vi "Fluke7320.vi"() -> ()   [LabVIEW 2017]
uses:
  <vilib>/Instr/_visa.llb/VISA Configure Serial Port (Instr).vi
panel:
  out "output cluster":cluster{dbl}={9.99}
  in  "Tab Control":enum32{"Com Settings", "File"}(tab)
  in  "VISA resource name":refnum<visa-resource-name>="COM28"
  in  "baud rate 2":u32=2400
  in  "base path":path=path "E:/Materials Testing"
  in  "Filename":string="Run1_Fluke"
  out "file path":path=path "E:/Materials Testing/2018-04-16/Run4_Fluke.tdms"
  out "XY Graph":cluster{timestamp[], dbl[]}(graph)={[timestamp(3606762406.9225206 s since 1904-01-01)], [9.99]}
  out "Current Set":string="set:   10.00 C\r"
  in  "Update set?":bool
  in  "Set to":dbl=20.0 format="%#_13g"
  out "Heater Power":string="po:   20\r"
  out "Temperature":string="t:    9.99 C\r"
  out "error out":errorcluster
  in  "error in (no error)":errorcluster
  in  "Stop":bool
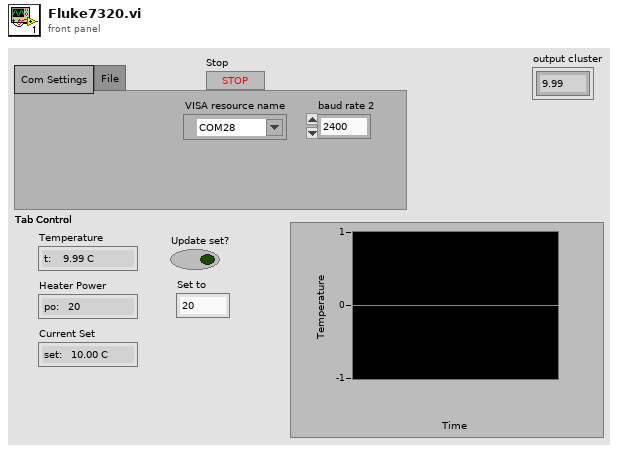
[diagram p1: front panel]
types:
  T1 = enum16{"open", "open or create", "create or replace", "create", "open (read-only)"}
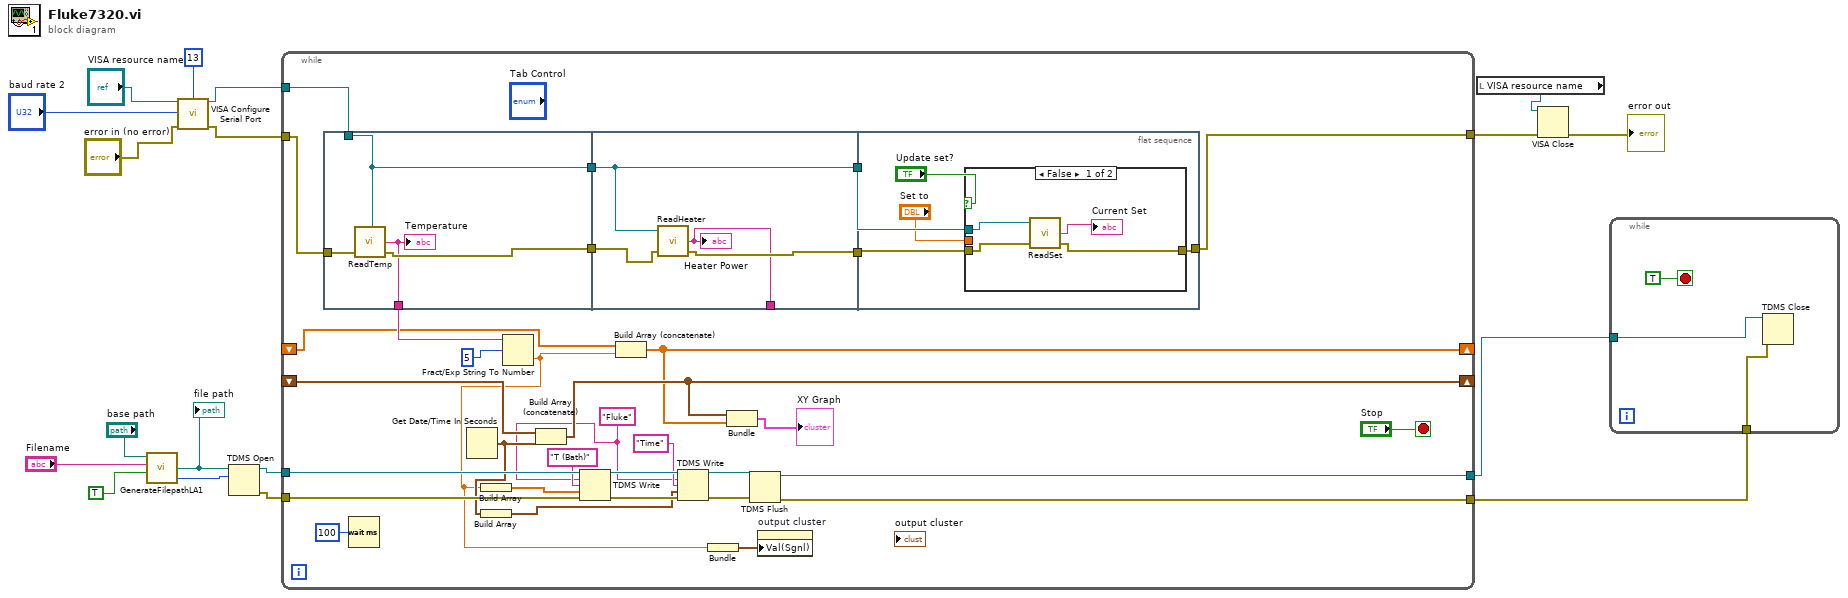
[diagram p0: block diagram]
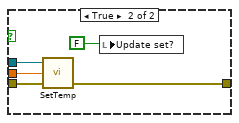
[diagram p2: hidden frame]
diagram:
  n1 = call "GenerateFilepathLA1.vi"("Auto Date folder"=TRUE, "Filename"="Filename", "base path"="base path") -> ("operation (0:open)"=w6:T1, "file path"=w5:path)  [unwired: 1 in, 1 out]
  "file path" <- w5
  n2 = call-poly "VISA Configure Serial Port"("VISA resource name"="VISA resource name", "termination char\n(0xA = '\\n' = LF)"=u8 13 ("termination char\n(0xA = '\\n' = LF)"), "baud rate (9600)"="baud rate 2", "error in (no error)"="error in (no error)") -> ("VISA resource name out"=w15:refnum<visa-resource-name>, "error out"=w14:errorcluster)  [unwired: 10 in]
  n3 = TDMS Open(10:w6, 11:w5) -> (0:w3:errorcluster, 3:w4:refnum<k34>)  [unwired: 5 in]
  n4 = while {
    tunnel: w14 -> [w48]
    tunnel: w15 -> [w47]
    tunnel: [w42] -> w10
    shift-right: [w36] -> _
    shift-left: _ -> [w39]
    shift-right: [w37] -> _
    shift-left: _ -> [w38]
    tunnel: w4 -> [w33]
    tunnel: w3 -> [w32]
    tunnel: [w25] -> w2
    tunnel: [w24] -> w1
    stop <- "Stop" stop-if-true
    w21 = "Fluke"
    n5 = flat-sequence {
      tunnel: w48 -> [w54]
      tunnel: w47 -> [w53]
      tunnel: [w53] -> w46
      tunnel: [w52] -> w45
      tunnel: [w51] -> w40
      tunnel: [w56] -> w44
      tunnel: w46 -> [w58]
      tunnel: [w58] -> w43
      tunnel: w45 -> [w57]
      tunnel: [w55] -> _
      tunnel: w44 -> [w63]
      tunnel: w43 -> [w62]
      tunnel: [w60] -> w42
      frame #0 {
        n6 = call "ReadTemp.vi"("error in (no error)"=w54, "VISA resource name"=w53) -> ("error out"=w52:errorcluster, "Temperature"=w51:string)  [unwired: 2 in]
        "Temperature" <- w51
      }
      frame #1 {
        n7 = call "ReadHeater.vi"("error in (no error)"=w57, "VISA resource name"=w58) -> ("error out"=w56:errorcluster, "Power"=w55:string)  [unwired: 1 in, 1 out]
        "Heater Power" <- w55
      }
      frame #2 {
        n8 = case shown="False" "Update set?" {
          tunnel: w63 -> [w66 w72]
          tunnel: [w65 w71] -> w60
          tunnel: w62 -> [w67 w70]
          tunnel: "Set to" -> [_ w69]
          frame False {
            n9 = call "ReadSet.vi"("error in (no error)"=w66, "VISA resource name"=w67) -> ("error out"=w65:errorcluster, "Set Temperature"=→"Current Set":string)  [unwired: 2 in]
          }
          frame True {
            n10 = call "SetTemp.vi"("error in (no error)"=w72, "Set Temperature"=w69, "VISA resource name"=w70) -> ("error out"=w71:errorcluster)  [unwired: 2 in]
            n11 = local write "Update set?"(FALSE) -> ()
          }
        }
      }
    }
    n12 = Wait (ms)(milliseconds to wait=u32 100) -> ()  [unwired: 1 out]
    n13 = Get Date/Time In Seconds() -> (seconds since 1Jan1904=w29:timestamp)
    n14 = Build Array(w29) -> (w28:timestamp[])
    n15 = Fract/Exp String To Number(string=w40, offset=5) -> (number=w20:dbl)  [unwired: 2 in, 1 out]
    n16 = Build Array(w20) -> (w34:dbl[])
    n17 = Build Array (concatenate)(w38, w29) -> (w37:timestamp[])
    n18 = TDMS Write(0:w33, 5:w21, 7:"T (Bath)", 9:w34, 11:w32) -> (4:w31:refnum<k34>, 15:w30:errorcluster)  [unwired: 1 in, 2 out]
    n19 = Build Array (concatenate)(w39, w20) -> (w36:dbl[])
    n20 = TDMS Write(0:w31, 5:w21, 7:"Time", 9:w28, 11:w30) -> (4:w26:refnum<k34>, 15:w27:errorcluster)  [unwired: 1 in, 2 out]
    n21 = Bundle(w20) -> (w19:cluster{dbl})  [unwired: 1 in]
    n22 = Bundle(w37, w36) -> (→"XY Graph":cluster{timestamp[], dbl[]})  [unwired: 1 in]
    n23 = TDMS Flush(4:w27, 7:w26) -> (0:w24:errorcluster, 3:w25:refnum<k34>)
    n24 = property on="output cluster" class="Clust (strict)"("Val(Sgnl)"=w19) -> ()  [unwired: 2 in, 2 out]
  }
  n25 = local read "VISA resource name"() -> (w11:refnum<visa-resource-name>)
  n26 = VISA Close(VISA resource name=w11, error in (no error)=w10) -> (error out=→"error out":errorcluster)
  n27 = while {
    tunnel: w2 -> [w73]
    tunnel: w1 -> [w74]
    stop <- TRUE stop-if-true
    n28 = TDMS Close(8:w74, 11:w73) -> ()  [unwired: 2 out]
  }
